vi "AlliGator FMB Global.vi"() -> ()   [LabVIEW 2021, in "AlliGator Fit Method Benchmark.lvlib"]
uses:
  AlliGator Fit Method Benchmark.lvlib
panel:
  out "Abort":bool
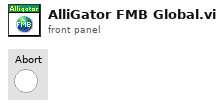
[diagram p1: front panel]
diagram:
